vi "User Updated Status.vi"(8 "error in (no error)":errorcluster, 10 "Status":string, 11 "Chat Window Model in":refnum<class "Chat Window Model.lvclass">) -> (0 "error out":errorcluster, 3 "Chat Window Model out":refnum<class "Chat Window Model.lvclass">)   [LabVIEW 2020, in "Chat Window Model.lvlib" / "Chat Window Model.lvclass"]
uses:
  Chat Window Model.lvclass
  C:/Program Files/National Instruments/LabVIEW 2020/vi.lib/ActorFramework/Actor/Actor.lvclass
  Event-Source-Actor/Data Interface/Status Data/Status Data.lvclass
  C:/Users/huipeng8/Desktop/SubPanel-Actor-Framework-master/Event-Source-Actor/Source/Template Source/Event Data/Event Data.lvclass
  <vilib>/ActorFramework/Actor/Actor.lvclass/Actor.ctl
  <vilib>/ActorFramework/Message Enqueuer/Message Enqueuer.lvclass/Message Enqueuer.ctl
  Chat Window Model.lvclass/Chat Window Model.ctl
  SubPanel-Actor-Framework-master/Event-Source-Actor/Source/Template Source/Event Source Messages/Generate Event Msg/Generate Event Msg.lvclass/Generate Event Msg.ctl
  Chat Window UI Controller/Chat Window UI Controller Messages/Update VI Title Msg/Update VI Title Msg.lvclass/Update VI Title Msg.ctl
  <vilib>/ActorFramework/Message Enqueuer/Init from Existing Queue.vi
  <vilib>/ActorFramework/Message Enqueuer/Enqueue.vi
  Chat Window UI Controller/Chat Window UI Controller Messages/Update VI Title Msg/Update VI Title Msg.lvclass
  C:/Program Files/National Instruments/LabVIEW 2020/vi.lib/ActorFramework/Message/Message.lvclass
  SubPanel-Actor-Framework-master/Event-Source-Actor/Source/Template Source/Event Source Messages/Generate Event Msg/Generate Event Msg.lvclass
  <vilib>/ActorFramework/Message Priority Queue/Priority Enqueue.vi
  <vilib>/ActorFramework/Message Enqueuer/Message Enqueuer.lvclass
  <vilib>/ActorFramework/Actor/Actor.lvclass
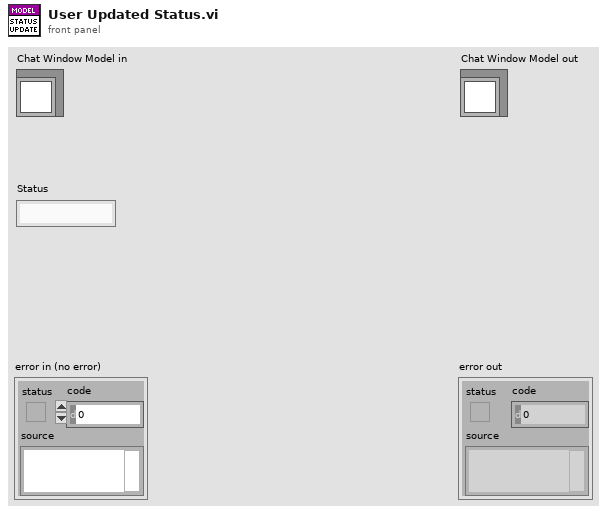
[diagram p1: front panel]
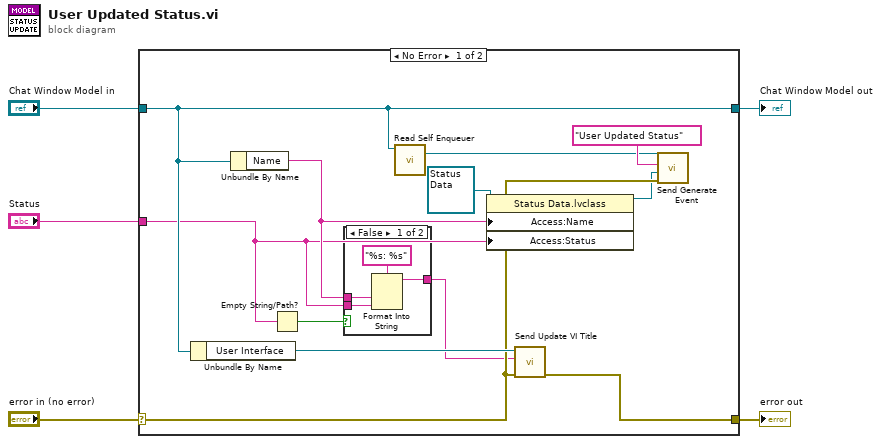
[diagram p0: block diagram]
diagram:
  n1 = case shown="No Error" "error in (no error)" {
    selector: "error in (no error)" -> [w11 w24]
    tunnel: [w15 w24] -> w4
    tunnel: [w14 w23] -> w2
    tunnel: "Chat Window Model in" -> [w14 w23]
    tunnel: "Status" -> [w6 _]
    frame No Error {
      n2 = Unbundle By Name(w14) -> ("User Interface"=w17:refnum<class "Message Enqueuer.lvclass">)
      n3 = Unbundle By Name(w14) -> ("Name"=w7:string)
      n4 = Empty String/Path?(string/path=w6) -> (empty?=w16:bool)
      n5 = case shown="False" w16 {
        tunnel: [w20 w22] -> w9
        tunnel: w7 -> [w19 w22]
        tunnel: w6 -> [w18 _]
        frame False {
          n6 = Format Into String(format string="%s: %s", w19, w18) -> (resulting string=w20:string)  [unwired: 2 in, 1 out]
        }
        frame True {
        }
      }
      n7 = call <vilib>:"Read Self Enqueuer.vi"("Actor"=w14) -> ("Self Enqueuer"=w12:refnum<class "Message Enqueuer.lvclass">)  [unwired: 10 in]
      n8 = property class="Status Data.lvclass"(reference=refnum<class "Status Data.lvclass"> refnum ("Status Data.lvclass"), "Access:Name"=w7, "Access:Status"=w6) -> (reference out=w8:refnum<class "Status Data.lvclass">)  [unwired: 1 in, 1 out]
      n9 = call "Send Update VI Title.vi"("error in (no error)"=w11, "Window Title"=w9, "Message Enqueuer in"=w17) -> ("error out"=w15:errorcluster)  [unwired: 7 in, 1 out]
      n10 = call "Send Generate Event.vi"("error in"=w11, "Event Data"=w8, "Event Name"="User Updated Status", "Message Enqueuer"=w12) -> ()  [unwired: 6 in, 2 out]
    }
    frame Error {
    }
  }
  "error out" <- w4
  "Chat Window Model out" <- w2
